vi "WLAN - QCA - UUT - AutoTest.vi"() -> ()   [LabVIEW 2011]
uses:
  niWLAN/WLAN -  niWLAN - INC - Select Measurement.ctl
  <userlib>/niRF/niSystem/SA/Includes/niSYS - SA - INC - STYP - Trigger.ctl
  <userlib>/niRF/niSystem/SA/Includes/niSYS - SA - INC - STYP - Trigger Delay.ctl
  Calibrate NART DUT Example Folder/ART2 Test Panel/LVx Folder/Support/TypeDef/TX Cal Data Rate.ctl
panel:
  in  "OTP":bool
  in  "NI HW":bool=TRUE
  in  "Calibration Folder Path":path=path "C:/LVProject_Dll/WLAN Reference/System Calibration"
  in  "Calibrate TX of DUT?":bool
  out "Total RX Time (ms)":u32=43271
  out "Total TX Time (ms)":u32=5562
  out "Total Cal Time (ms)":u32
  out "Total Init Time (ms)":u32=11744
  out "Total Test Time (ms)":u32=60599
  out "error out":errorcluster
  in  "nart directory":path=path "C:/Users/ni/Desktop/art2_ver_2_28_6BIN/bin"
  in  "Select Standard":T1={"Tx_ 802.11a/g OFDM"=TRUE, "Tx_ 802.11b DSSS/CCK"=FALSE, "Tx_ 802.11n OFDM "=TRUE, "Tx_ 802.11ac OFDM "=FALSE}
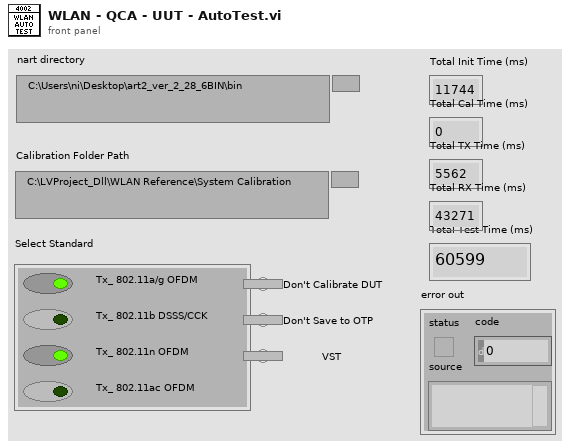
[diagram p1: front panel]
types:
  T1 = typedef "WLAN -  niWLAN - INC - Select Measurement.ctl" = cluster{"Tx_ 802.11a/g OFDM":bool, "Tx_ 802.11b DSSS/CCK":bool, "Tx_ 802.11n OFDM ":bool, "Tx_ 802.11ac OFDM ":bool}
  T2 = typedef "TX Cal Data Rate.ctl" = cluster{"Frequency":u32, "TX Gain":u32, "LL":i32, "UL":u32}
  T3 = typedef "niSYS - SA - INC - STYP - Trigger.ctl" = cluster{"Source":enum16{"Immediate", "External", "Software", "RTSI 0", "RTSI 1", "RTSI 2", "RTSI 3", "RTSI 4", "RTSI 5", "RTSI 6", "RTSI 7", "PFI 0", "PFI 1", "PFI 2", "PXI Star", "Power"}, "Edge":enum16{"Rising", "Falling"}, "Delay, sec":T4, "Level, dBm":dbl, "Min Quiet Time, sec":dbl}
  T4 = typedef "niSYS - SA - INC - STYP - Trigger Delay.ctl" = dbl
  T5 = cluster{"Temperature, C":dbl, "Time Stamp, sec":dbl, "Calibration Table":dbl[][]}
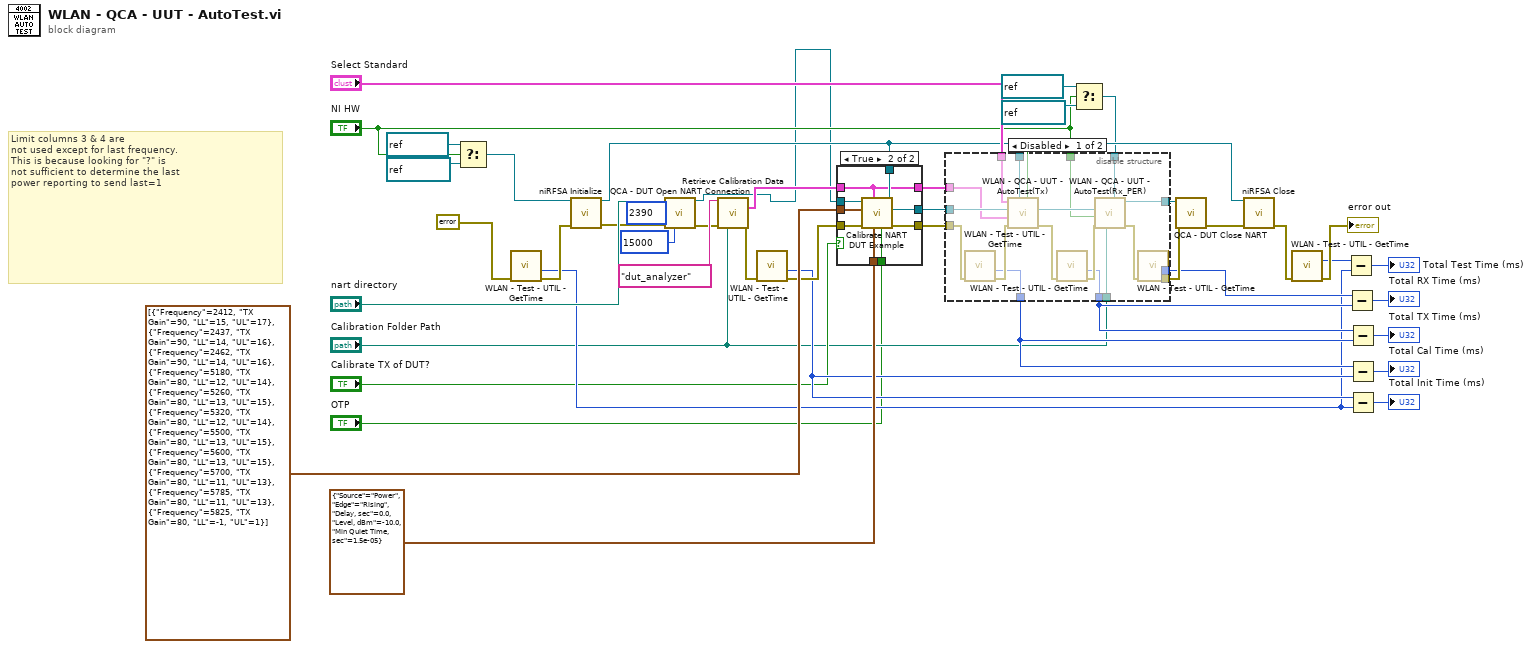
[diagram p0: block diagram]
diagram:
  # "Limit columns 3 & 4 are\nnot used except for last frequency.\nThis is because looking for \"?\" is\nnot sufficient to determine the last\npower reporting to send last=1"
  n1 = Select(t=refnum<k15> "RIO0" ("resource name"), s="NI HW", f=refnum<k15> "RFSA" ("resource name")) -> (s? t:f=w4:refnum<k15>)
  n2 = call "WLAN - Test - UTIL - GetTime.vi"("error in (no error)"=errorcluster {"status"=FALSE, "code"=0, "source"=""}) -> ("error out"=w33:errorcluster, "millisecond timer value"=w19:u32)  [unwired: 8 in, 1 out]
  n3 = call <instrlib>:"niRFSA Initialize.vi"("resource name"=w4, "error in"=w33) -> ("instrument handle"=w36:refnum<k15>, "error out"=w37:errorcluster)  [unwired: 12 in]
  n4 = call "QCA - DUT Open NART Connection.vi"("NART Directory"="nart directory", "port (2390)"=u32 2390, "error in (no error)"=w37, "Timeout (2500ms)"=15000) -> ("NART TCP Connection"=w1:refnum<k5>, "error out"=w14:errorcluster)  [unwired: 10 in]
  n5 = call "Retrieve Calibration Data.vi"("Calibration Signal Path Name"="dut_analyzer", "error in (no error)"=w14, "Folder Path"="Calibration Folder Path") -> ("Calibration Data"=w12:T5, "error out"=w13:errorcluster)  [unwired: 11 in]
  n6 = call "WLAN - Test - UTIL - GetTime.vi"("error in (no error)"=w13) -> ("error out"=w31:errorcluster, "millisecond timer value"=w20:u32)  [unwired: 8 in, 1 out]
  n7 = case shown="True" "Calibrate TX of DUT?" {
    tunnel: T3 {"Source"=enum."Power", "Edge"=enum."Rising", "Delay, sec"=0.0, "Level, dBm"=-10.0, "Min Quiet Time, sec"=1.5e-05} ("Trigger") -> [_ w57]
    tunnel: w1 -> [w47 w56]
    tunnel: [w47 w55] -> w39
    tunnel: w36 -> [_ w54]
    tunnel: T2[] [{"Frequency"=2412, "TX Gain"=90, "LL"=15, "UL"=17}, {"Frequency"=2437, "TX Gain"=90, "LL"=14, "UL"=16}, {"Frequency"=2462, "TX Gain"=90, "LL"=14, "UL"=16}, {"Frequency"=5180, "TX Gain"=80, "LL"=12, "UL"=14}, {"Frequency"=5260, "TX Gain"=80, "LL"=13, "UL"=15}, {"Frequency"=5320, "TX Gain"=80, "LL"=12, "UL"=14}, {"Frequency"=5500, "TX Gain"=80, "LL"=13, "UL"=15}, {"Frequency"=5600, "TX Gain"=80, "LL"=13, "UL"=15}, {"Frequency"=5700, "TX Gain"=80, "LL"=11, "UL"=13}, {"Frequency"=5785, "TX Gain"=80, "LL"=11, "UL"=13}, {"Frequency"=5825, "TX Gain"=80, "LL"=-1, "UL"=1}] ("Frequency and Tx Gain") -> [_ w53]
    tunnel: w31 -> [w48 w52]
    tunnel: [w48 w51] -> w30
    tunnel: w12 -> [w46 w50]
    tunnel: [w46 w50] -> w11
    tunnel: "OTP" -> [_ w49]
    frame False {
    }
    frame True {
      n8 = call "Calibrate NART DUT Example.vi"("RFSA Handle In"=w54, "OTP"=w49, "Trigger"=w57, "Calibration Data"=w50, "error in (no error)"=w52, "Frequency and Tx Gain"=w53, "CART TCP Connection In"=w56) -> ("error out"=w51:errorcluster, "CART TCP Connection Out"=w55:refnum<k5>)  [unwired: 3 in]
    }
  }
  n9 = Select(t=refnum<k15> "RIO0" ("VSG Resource Name"), s="NI HW", f=refnum<k15> "RFSG" ("VSG Resource Name")) -> (s? t:f=w7:refnum<k15>)
  n10 = disable-structure shown="Disabled" {
    disable-tunnel: "Select Standard" -> [w75 _]
    disable-tunnel: [w73 w76] -> w40
    disable-tunnel: w39 -> [w72 w76]
    disable-tunnel: w36 -> [w71 _]
    disable-tunnel: w30 -> [w70 _]
    disable-tunnel: [w65 _] -> w29
    disable-tunnel: [w64 _] -> w23
    disable-tunnel: [w63 _] -> w22
    disable-tunnel: [w62 _] -> w21
    disable-tunnel: w11 -> [w61 _]
    disable-tunnel: "Calibration Folder Path" -> [w60 _]
    disable-tunnel: w7 -> [w59 _]
    disable-tunnel: "NI HW" -> [w58 _]
    frame Disabled {
      n11 = call "WLAN - Test - UTIL - GetTime.vi"("error in (no error)"=w70) -> ("error out"=w69:errorcluster, "millisecond timer value"=w62:u32)  [unwired: 8 in, 1 out]
      n12 = call "WLAN - QCA - UUT - AutoTest(Tx).vi"("NI HW"=w58, "RFSA"=w71, "error in (no error)"=w69, "Calibration Data"=w61, "NART TCP Connection"=w72, "Select Standard"=w75) -> ("error out"=w68:errorcluster, "NART TCP Connection Out"=w74:refnum<k5>)  [unwired: 4 in]
      n13 = call "WLAN - Test - UTIL - GetTime.vi"("error in (no error)"=w68) -> ("error out"=w67:errorcluster, "millisecond timer value"=w63:u32)  [unwired: 8 in, 1 out]
      n14 = call "WLAN - QCA - UUT - AutoTest(Rx_PER).vi"("VSG Resource Name"=w59, "Calibration Folder Path"=w60, "error in (no error)"=w67, "NI HW"=w58, "NART TCP Connection"=w74) -> ("error out"=w66:errorcluster, "CART TCP Connection Out"=w73:refnum<k5>)  [unwired: 5 in]
      n15 = call "WLAN - Test - UTIL - GetTime.vi"("error in (no error)"=w66) -> ("error out"=w65:errorcluster, "millisecond timer value"=w64:u32)  [unwired: 8 in, 1 out]
    }
    frame Enabled {
    }
  }
  n16 = call "QCA - DUT Close NART.vi"("CART TCP Connection"=w40, "error in (no error)"=w29) -> ("error out"=w38:errorcluster)  [unwired: 13 in]
  n17 = call <instrlib>:"niRFSA Close.vi"("instrument handle"=w36, "error in"=w38) -> ("error out"=w28:errorcluster)  [unwired: 13 in]
  n18 = call "WLAN - Test - UTIL - GetTime.vi"("error in (no error)"=w28) -> ("error out"=→"error out":errorcluster, "millisecond timer value"=w24:u32)  [unwired: 8 in, 1 out]
  n19 = Subtract(x=w24, y=w19) -> (x-y=→"Total Test Time (ms)":u32)
  n20 = Subtract(x=w23, y=w22) -> (x-y=→"Total RX Time (ms)":u32)
  n21 = Subtract(x=w22, y=w21) -> (x-y=→"Total TX Time (ms)":u32)
  n22 = Subtract(x=w21, y=w20) -> (x-y=→"Total Cal Time (ms)":u32)
  n23 = Subtract(x=w20, y=w19) -> (x-y=→"Total Init Time (ms)":u32)
